vi "Create Attribute.vi"   [LabVIEW 2020, in "VILab.lvlib" / "Attribute.lvclass"]
uses:
  Attribute.lvclass
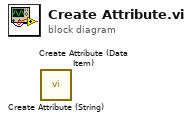
[diagram p0: block diagram]
diagram:
  n1 = call "Create Attribute (String).vi"() -> ()  [unwired: 11 in, 1 out]
  n2 = call "Create Attribute (Data Item).vi"() -> ()  [unwired: 11 in, 1 out]
